vi "To String Array.vi"(8 "error in (no error)":errorcluster, 11 "Numeric Limit Compare Config in":refnum<class "Numeric Limit Compare Config.lvclass">) -> (0 "error out":errorcluster, 1 "Step String Array":string[](array[string]), 3 "Numeric Limit Compare Config out":refnum<class "Numeric Limit Compare Config.lvclass">)   [LabVIEW 2015, in "Numeric Limit Compare Config.lvclass"]
uses:
  Numeric Limit Compare Config.lvclass
  Numeric Limit Compare Config.lvclass/Numeric Limit Compare Config.ctl
  <vilib>/NI/Tag Bus/tag/tag descriptor.lvclass/tag descriptor.ctl
  Read Channel.vi
  Read Comparison Type.vi
  Read Negate Result.vi
  Read Upper Limit_Limit.vi
  Read Lower Limit.vi
  classes/Step/Config/Step Config.lvclass
  <vilib>/NI/Tag Bus Module Framework/channel/TBM channel.lvclass
  <vilib>/NI/Tag Bus/tag/tag descriptor.lvclass
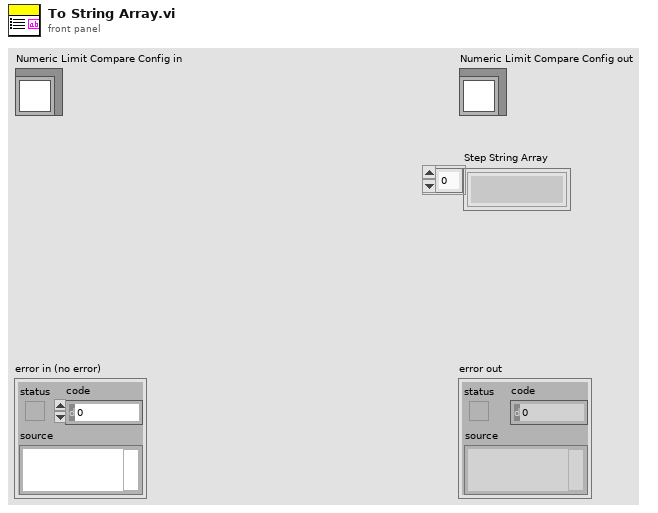
[diagram p1: front panel]
types:
  T1 = typedef "Comparison Types.ctl" = enum16{"GELE (>=<=)", "GTLE(><=)", "GTLT(><)", "GELT(>=<)", "EQ(==)", "NE (!=)", "GT(>)", "LT(<)", "GE(>=)", "LE(<=)"}
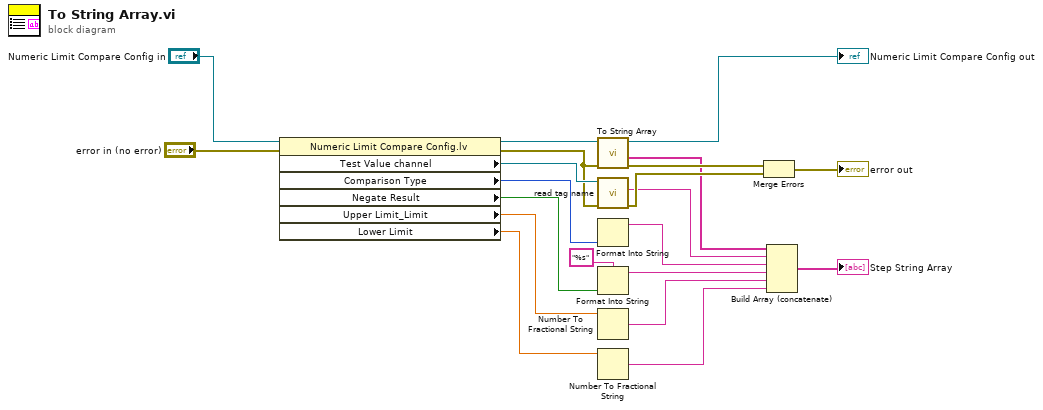
[diagram p0: block diagram]
diagram:
  n1 = property class="Numeric Limit Compare Config.lv"(reference="Numeric Limit Compare Config in", error in="error in (no error)") -> (reference out=w19:refnum<class "Numeric Limit Compare Config.lvclass">, error out=w14:errorcluster, "Test Value channel"=w16:refnum<class "TBM channel.lvclass">, "Comparison Type"=w15:T1, "Negate Result"=w8:bool, "Upper Limit_Limit"=w13:dbl, "Lower Limit"=w12:dbl)
  n2 = call-parent "To String Array.vi"("error in (no error)"=w14, "Step Config in"=w19) -> ("error out"=w9:errorcluster, "Step String Array"=w7:string[], "Step Config out"=→"Numeric Limit Compare Config out":refnum<class "Numeric Limit Compare Config.lvclass">)  [unwired: 7 in]
  n3 = call <vilib>:"read tag name.vi"("error in"=w14, "system tag in"=w16) -> ("error out"=w10:errorcluster, "name"=w6:string)  [unwired: 7 in, 1 out]
  n4 = Format Into String(w15) -> (resulting string=w5:string)  [unwired: 3 in, 1 out]
  n5 = Format Into String(format string="%s", w8) -> (resulting string=w4:string)  [unwired: 2 in, 1 out]
  n6 = Number To Fractional String(number=w13) -> (F-format string=w3:string)  [unwired: 3 in]
  n7 = Number To Fractional String(number=w12) -> (F-format string=w2:string)  [unwired: 3 in]
  n8 = Merge Errors(w9, w10) -> (→"error out":errorcluster)
  n9 = Build Array (concatenate)(w7, w6, w5, w4, w3, w2) -> (→"Step String Array":string[])
